vi "Overlay Images.vi"(0 "image in":refnum<class "MSC Image.lvclass">, 1 "image 2 in":refnum<class "MSC Image.lvclass">, 2 "alpha":dbl=0.5, 3 "beta":dbl=0.5, 5 "error in (no error)":errorcluster) -> (14 "image out":refnum<class "MSC Image.lvclass">, 15 "image 2 out":refnum<class "MSC Image.lvclass">, 19 "error out":errorcluster)   [LabVIEW 2014, in "MSC Image.lvclass"]
doc: "Overlays two images.\n\nimage = (alpha * image) + (beta * image 2)"
uses:
  MSC Image.lvclass
  MSC Image.lvclass/MSC Image.ctl
  Dependencies/x86/MSC I Process32.dll
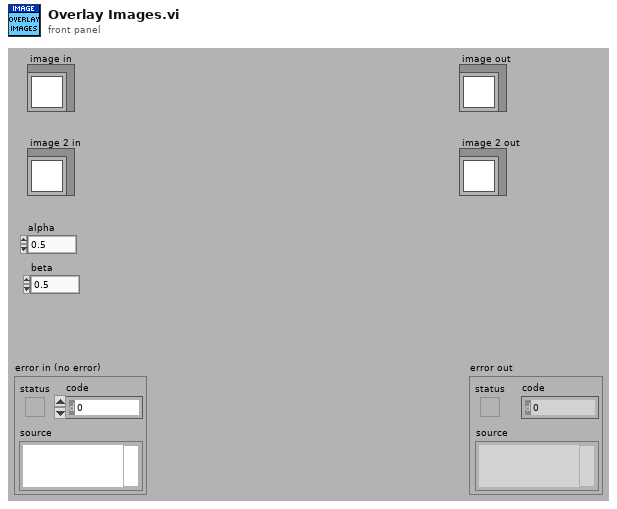
[diagram p1: front panel]
types:
  T1 = typedef "Image.ctl" = cluster{"Pointer":u64, "Size":T2, "Image Type":T3, "Time Stamp":timestamp, "Variant":variant}
  T2 = typedef "Size.ctl" = cluster{"Cols":i32, "Rows":i32}
  T3 = typedef "Image Type.ctl" = i32
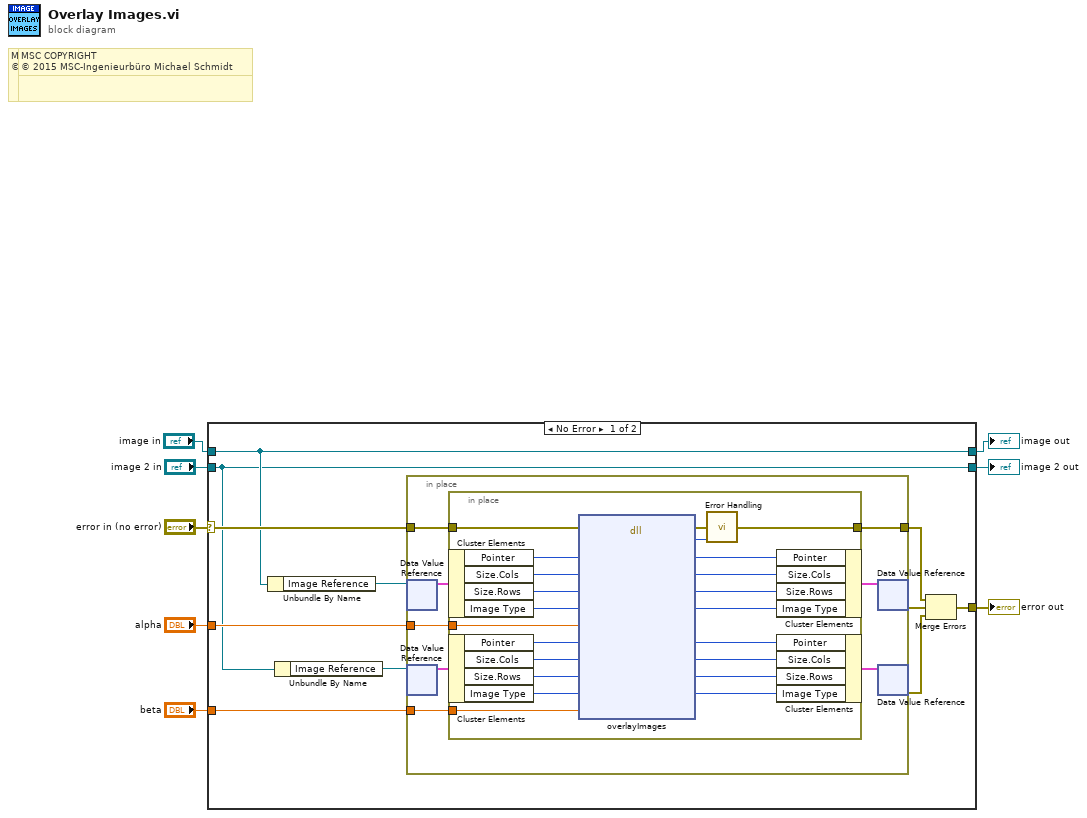
[diagram p0: block diagram]
diagram:
  # "MSC COPYRIGHT\n© 2016 MSC-Ingenieurbüro Michael Schmidt"
  # "MSC COPYRIGHT\n© 2016 MSC-Ingenieurbüro Michael Schmidt"
  # "MSC COPYRIGHT\n© 2015 MSC-Ingenieurbüro Michael Schmidt"
  # "MSC COPYRIGHT\n© 2015 MSC-Ingenieurbüro Michael Schmidt"
  n1 = case shown="No Error" "error in (no error)" {
    selector: "error in (no error)" -> [w13 w52]
    tunnel: [w19 w52] -> w4
    tunnel: [w9 w51] -> w7
    tunnel: "image in" -> [w12 w50]
    tunnel: "image 2 in" -> [w9 w51]
    tunnel: [w12 w50] -> w8
    tunnel: "alpha" -> [w15 _]
    tunnel: "beta" -> [w14 _]
    frame No Error {
      n2 = Unbundle By Name(w12) -> ("Image Reference"=w11:refnum<data-value>)
      n3 = Unbundle By Name(w9) -> ("Image Reference"=w10:refnum<data-value>)
      n4 = in-place {
        in-place-border: w13 -> [w25]
        in-place-border: [w24] -> w18
        in-place-border: w15 -> [w21]
        in-place-border: w14 -> [w20]
        n5 = in-place-dvr #1(w11) -> (w26:T1)  [unwired: 1 out]
        n6 = in-place-dvr #2(w10) -> (w23:T1)  [unwired: 1 out]
        n7 = in-place {
          in-place-border: w25 -> [w30]
          in-place-border: [w49] -> w24
          in-place-border: w21 -> [w29]
          in-place-border: w20 -> [w28]
          n8 = in-place-cluster #3(w26) -> ("Pointer"=w48:u64, "Size.Cols"=w47:i32, "Size.Rows"=w46:i32, "Image Type"=w45:T3)
          n9 = in-place-cluster #4(w23) -> ("Pointer"=w44:u64, "Size.Cols"=w43:i32, "Size.Rows"=w42:i32, "Image Type"=w41:T3)
          n10 = dll-call lib="C:/Users/MSC/LabVIEW Projekte/LV 2014/MSC I-Process/user.lib/MSC-I Process/Dependencies/x86/MSC I Process*.dll" fn="overlayImages"(error in=w30, "pointer"=w48, "cols"=w47, "rows"=w46, "type"=w45, "alpha"=w29, "pointer2"=w44, "cols2"=w43, "rows2"=w42, "type2"=w41, "beta"=w28) -> (error out=w31:errorcluster, "error"=w32:i32, "pointer"=w36:u64, "cols"=w35:i32, "rows"=w34:i32, "type"=w33:i32, "pointer2"=w40:u64, "cols2"=w39:i32, "rows2"=w38:i32, "type2"=w37:i32)  [unwired: 4 in, 1 out]
          n11 = call "Error Handling.vi"("error in (no error)"=w31, "return type"=w32) -> ("error out"=w49:errorcluster)  [unwired: 12 in, 1 out]
          n12 = in-place-cluster #3("Pointer"=w36, "Size.Cols"=w35, "Size.Rows"=w34, "Image Type"=w33) -> (w27:T1)
          n13 = in-place-cluster #4("Pointer"=w40, "Size.Cols"=w39, "Size.Rows"=w38, "Image Type"=w37) -> (w22:T1)
        }
        n14 = in-place-dvr #1(w27) -> (w17:errorcluster)  [unwired: 1 out]
        n15 = in-place-dvr #2(w22) -> (w16:errorcluster)  [unwired: 1 out]
      }
      n16 = Merge Errors(w18, w17, w16) -> (w19:errorcluster)
    }
    frame Error {
    }
  }
  "error out" <- w4
  "image out" <- w8
  "image 2 out" <- w7
